vi "Fetch Waveforms Means.vi"(8 "error in":errorcluster, 11 "Scope Base in":refnum<class "Scope Base.lvclass">) -> (0 "error out":errorcluster, 3 "Scope Base out":refnum<class "Scope Base.lvclass">)   [LabVIEW 2023]
uses:
  Scope Base.lvclass
  Interfaces/IConfigure Scope/IConfigure Scope.lvclass
  <vilib>/Analysis/NI_AALBase.lvlib
  <vilib>/ErrorRing/Error Ring.xnode
  <vilib>/Utility/error.llb/Error Cluster From Error Code.vi
  <vilib>/Analysis/baseanly.llb/Mean (DBL).vi
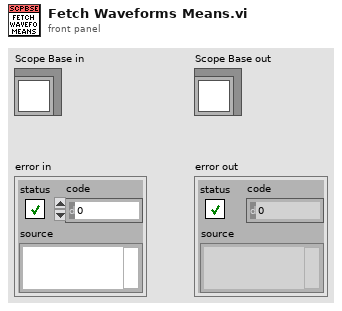
[diagram p1: front panel]
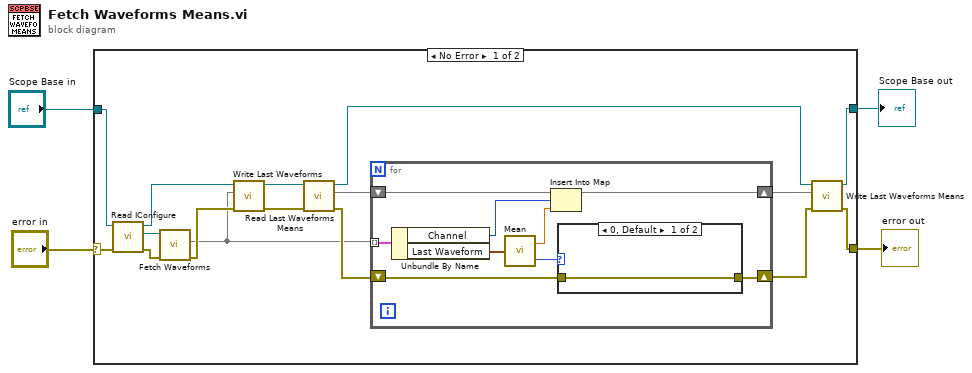
[diagram p0: block diagram]
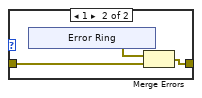
[diagram p2: hidden frame]
diagram:
  n1 = case shown="No Error" "error in" {
    selector: "error in" -> [w9 w40]
    tunnel: "Scope Base in" -> [w17 w39]
    tunnel: [w15 w40] -> w3
    tunnel: [w13 w39] -> w2
    frame No Error {
      n2 = call "Read IConfigure.vi"("error in (no error)"=w9, "Scope Base in"=w17) -> ("error out"=w19:errorcluster, "IConfigureScope"=w18:refnum<class "IConfigure.lvclass">, "Scope Base out"=w7:refnum<class "Scope Base.lvclass">)  [unwired: 7 in]
      n3 = call-dynamic "Fetch Waveforms.vi"("error in"=w19, "IConfigure Scope in"=w18) -> ("error out"=w20:errorcluster, "Last Waveforms"=w5:map{u8, waveform(dbl)})  [unwired: 7 in, 1 out]
      n4 = call "Write Last Waveforms.vi"("error in (no error)"=w20, "Last Waveforms"=w5, "Scope Base in"=w7) -> ("error out"=w8:errorcluster, "Scope Base out"=w6:refnum<class "Scope Base.lvclass">)  [unwired: 7 in]
      n5 = call-dynamic "Read Last Waveforms Means.vi"("error in (no error)"=w8, "Scope Base in"=w6) -> ("error out"=w12:errorcluster, "Last Waveforms Means"=w16:map{u8, dbl}, "Scope Base out"=w14:refnum<class "Scope Base.lvclass">)  [unwired: 7 in]
      n6 = for {
        tunnel: w5 -> [w28] mode=indexing
        shift-right: [w24] -> w11
        shift-left: w16 -> [w29]
        shift-right: [w21] -> w10
        shift-left: w12 -> [w22]
        n7 = Unbundle By Name(w28) -> ("Channel"=w27:u8, "Last Waveform"=w26:waveform(dbl))
        n8 = call-poly <vilib>:"Mean.vi"("X"=w26) -> ("mean"=w25:dbl, "error"=w23:i32)
        n9 = Insert Into Map(map in=w29, key=w27, value=w25) -> (map out=w24:map{u8, dbl})  [unwired: 2 out]
        n10 = case shown="0, Default" w23 {
          tunnel: w22 -> [w30 w33]
          tunnel: [w30 w32] -> w21
          frame 0, Default {
          }
          frame 1 {
            n11 = xnode "Error Ring"() -> ("error out"=w31:errorcluster)
            n12 = Merge Errors(w31, w33) -> (w32:errorcluster)
          }
        }
      }
      n13 = call "Write Last Waveforms Means.vi"("error in (no error)"=w10, "Last Voltage"=w11, "Scope Base in"=w14) -> ("error out"=w15:errorcluster, "Scope Base out"=w13:refnum<class "Scope Base.lvclass">)  [unwired: 7 in]
    }
    frame Error {
    }
  }
  "error out" <- w3
  "Scope Base out" <- w2
